vi "Write Buffer size.vi"(8 "error in (no error)":errorcluster, 10 "Buffer size":i32, 11 "Software Lock-in in":refnum<class "Software Lock-in.lvclass">) -> (0 "error out":errorcluster, 3 "Software Lock-in out":refnum<class "Software Lock-in.lvclass">)   [LabVIEW 2015, in "Software Lock-in.lvclass"]
uses:
  Software Lock-in.lvclass
  Software Lock-in.lvclass/Software Lock-in.ctl
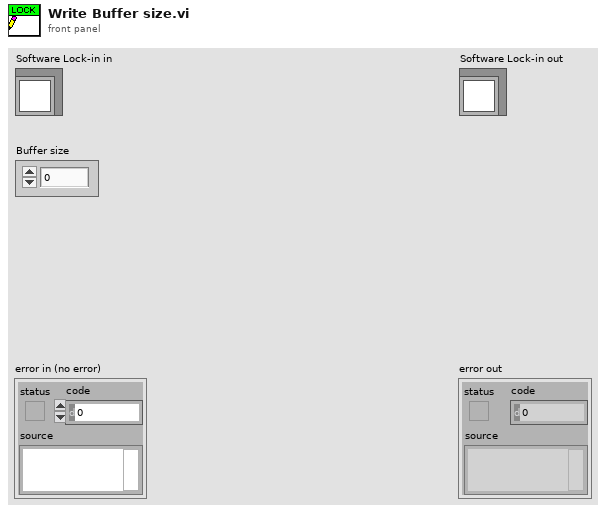
[diagram p1: front panel]
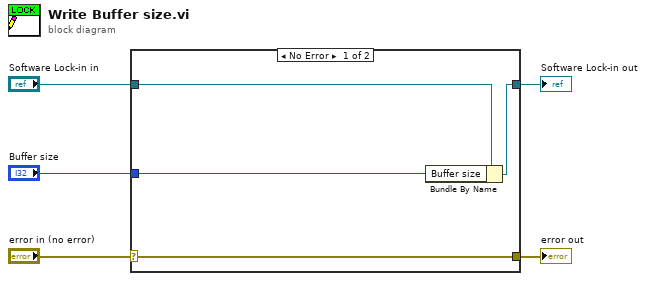
[diagram p0: block diagram]
diagram:
  n1 = case shown="No Error" "error in (no error)" {
    selector: "error in (no error)" -> [w9 w10]
    tunnel: [w9 w10] -> w4
    tunnel: [w7 w11] -> w2
    tunnel: "Software Lock-in in" -> [w8 w11]
    tunnel: "Buffer size" -> [w6 _]
    frame No Error {
      n2 = Bundle By Name(cluster=w8, "Buffer size"=w6) -> (w7:refnum<class "Software Lock-in.lvclass">)
    }
    frame Error {
    }
  }
  "error out" <- w4
  "Software Lock-in out" <- w2
